vi "Initialize.vi"(8 "error in":errorcluster, 10 "InstanceName":string, 11 "Chiller Cluster - 1 Channel.lvclass":refnum<class "Power Supply Cluster - 1 Channel.lvclass">) -> (0 "error out":errorcluster, 3 "output cluster":refnum<class "Power Supply Cluster - 1 Channel.lvclass">)   [LabVIEW 2023, in "Power Supply Cluster - 1 Channel.lvclass"]
uses:
  Power Supply Cluster - 1 Channel.lvclass
  Power Supply Cluster - 1 Channel.lvclass/Power Supply Cluster - 1 Channel.ctl
  546b7d5c-4f51-47af-9af1-567894f85656.vi
  397b3e0b-0f1b-47d9-9f6d-8a44e581e150.vi
  248f2659-eb42-462d-9a15-8e5b3aec119f.vi
  b9c13089-0281-44b9-a90f-aec73f88b65c.vi
  546b7d5c-4f51-47af-9af1-567894f85656.vi/4bc1c15b-36ab-481f-b8dd-c64075ce723a.vi
  397b3e0b-0f1b-47d9-9f6d-8a44e581e150.vi/4bc1c15b-36ab-481f-b8dd-c64075ce723a.vi
  248f2659-eb42-462d-9a15-8e5b3aec119f.vi/4bc1c15b-36ab-481f-b8dd-c64075ce723a.vi
  b9c13089-0281-44b9-a90f-aec73f88b65c.vi/4bc1c15b-36ab-481f-b8dd-c64075ce723a.vi
  <vilib>/ADAS Replay HIL/Channels/Tag Wrapper/Polymorphic/Open Consumer Tag (Cluster).vi
  <vilib>/ADAS Replay HIL/AdasHilServices/AdasHilServices Fill In Error Info Ex.vi
  <vilib>/ADAS Replay HIL/Channels/Tag Wrapper/Polymorphic/Open Producer Tag (Cluster).vi
  Utilities/Utilities.lvlib
  <vilib>/ADAS Replay HIL/Channels/Tag Wrapper/Tag Wrapper.lvlib
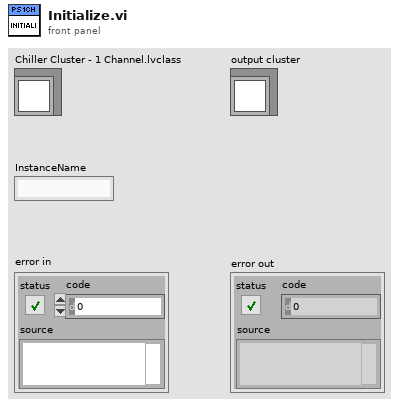
[diagram p1: front panel]
types:
  T1 = cluster{"OnOff.ACT":bool, "ErrorAcknowledge.ACT":bool}
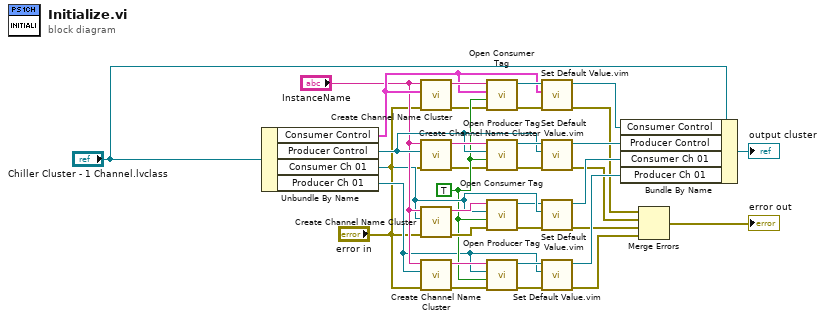
[diagram p0: block diagram]
diagram:
  w14 = TRUE ("Create if not found? (T)")
  n1 = Unbundle By Name("Chiller Cluster - 1 Channel.lvclass") -> ("Consumer Control"=w28:T1, "Producer Control"=w23:refnum<k21>, "Consumer Ch 01"=w18:refnum<k21>, "Producer Ch 01"=w13:refnum<k21>)
  n2 = call "Create Channel Name Cluster.vi"("error in"="error in", "Cluster"=w28, "Instance Name"="InstanceName") -> ("error out"=w7:errorcluster, "Data Channel Name"=w32:string)  [unwired: 7 in]
  n3 = call "Create Channel Name Cluster.vi"("error in"="error in", "Cluster"=w23, "Instance Name"="InstanceName") -> ("error out"=w8:errorcluster, "Data Channel Name"=w31:string)  [unwired: 7 in]
  n4 = call "Create Channel Name Cluster.vi"("error in"="error in", "Cluster"=w18, "Instance Name"="InstanceName") -> ("error out"=w15:errorcluster, "Data Channel Name"=w21:string)  [unwired: 7 in]
  n5 = call "Create Channel Name Cluster.vi"("error in"="error in", "Cluster"=w13, "Instance Name"="InstanceName") -> ("error out"=w11:errorcluster, "Data Channel Name"=w20:string)  [unwired: 7 in]
  n6 = call-poly <vilib>:"Open Consumer Tag.vi"("error in"=w7, "Create if not found? (T)"=w14, "Cluster"=w28, "Channel Name"=w32) -> ("error out"=w27:errorcluster, "ADAS HIL Channel"=w30:refnum<k21>)  [unwired: 6 in]
  n7 = call-poly <vilib>:"Open Producer Tag.vi"("error in"=w8, "Create if not found? (T)"=w14, "Cluster"=w23, "Channel Name"=w31) -> ("error out"=w26:errorcluster, "ADAS HIL Channel"=w25:refnum<k21>)  [unwired: 6 in]
  n8 = call-poly <vilib>:"Open Consumer Tag.vi"("error in"=w15, "Create if not found? (T)"=w14, "Cluster"=w18, "Channel Name"=w21) -> ("error out"=w16:errorcluster, "ADAS HIL Channel"=w17:refnum<k21>)  [unwired: 6 in]
  n9 = call-poly <vilib>:"Open Producer Tag.vi"("error in"=w11, "Create if not found? (T)"=w14, "Cluster"=w13, "Channel Name"=w20) -> ("error out"=w12:errorcluster, "ADAS HIL Channel"=w19:refnum<k21>)  [unwired: 6 in]
  n10 = call "Set Default Value.vim"("error in"=w27, "Data in"=w28, "ADAS HIL Channel in"=w30) -> ("error out"=w5:errorcluster, "ADAS HIL Channel out"=w29:refnum<k21>)  [unwired: 7 in]
  n11 = call "Set Default Value.vim"("error in"=w26, "Data in"=w23, "ADAS HIL Channel in"=w25) -> ("error out"=w4:errorcluster, "ADAS HIL Channel out"=w24:refnum<k21>)  [unwired: 7 in]
  n12 = call "Set Default Value.vim"("error in"=w16, "Data in"=w18, "ADAS HIL Channel in"=w17) -> ("error out"=w3:errorcluster, "ADAS HIL Channel out"=w10:refnum<k21>)  [unwired: 7 in]
  n13 = call "Set Default Value.vim"("error in"=w12, "Data in"=w13, "ADAS HIL Channel in"=w19) -> ("error out"=w2:errorcluster, "ADAS HIL Channel out"=w9:refnum<k21>)  [unwired: 7 in]
  n14 = Bundle By Name(cluster="Chiller Cluster - 1 Channel.lvclass", "Consumer Control"=w29, "Producer Control"=w24, "Consumer Ch 01"=w10, "Producer Ch 01"=w9) -> (→"output cluster":refnum<class "Power Supply Cluster - 1 Channel.lvclass">)
  n15 = Merge Errors(w5, w4, w3, w2) -> (→"error out":errorcluster)
